vi "OpenFiles.vi"() -> ()   [LabVIEW 2018]
uses:
  <vilib>/addons/h5labview2/file/H5Fmode.ctl
  HDF5/HDF5_NoiseInfoClust.ctl
  HDF5/lib_path_mod_20200519.vi
  <vilib>/addons/h5labview2/base/H5Equery.vi
  <vilib>/addons/h5labview2/dataset/H5Dread.llb/H5Dread.xnode
  <vilib>/addons/h5labview2/file/H5F.lvlib
  <vilib>/addons/h5labview2/group/H5G.lvlib
panel:
  in  "Tree":string(tree)
  out "Folders":path[](array[path])
  out "Groups":string[](array[string])
  in  "Select 2":bool
  in  "Listbox 2":i32[](listbox)
  in  "Select":bool
  in  "Listbox":i32[](listbox)
  out "filenames":string[](array[string])
  in  "path":path
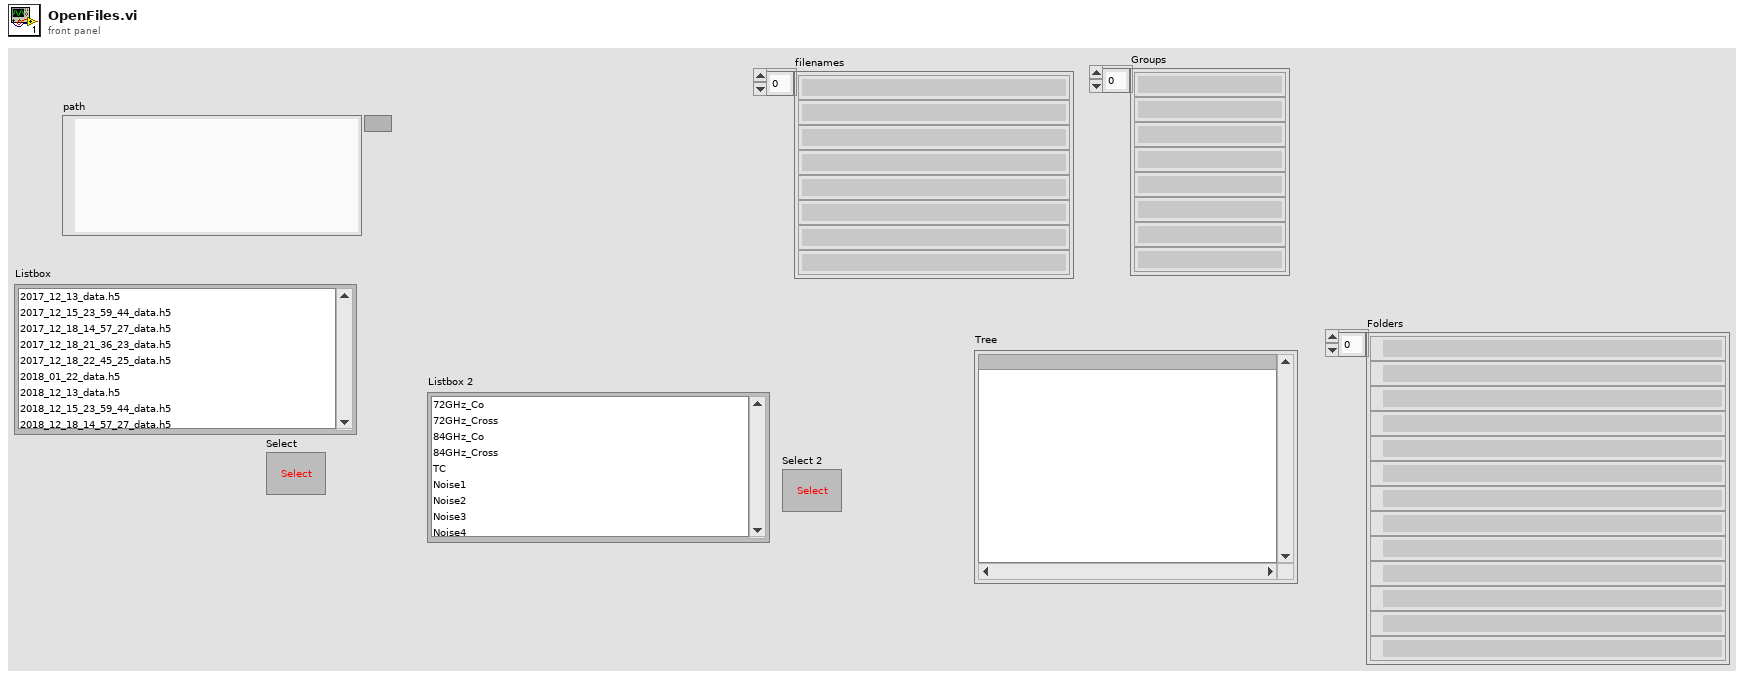
[diagram p1: front panel]
types:
  T1 = typedef "H5F.lvlib/H5Fmode.ctl" = enum16{"read-only", "read-write", "overwrite", "create new", "open or create"}
  T2 = typedef "hid_t.ctl" = i32
  T3 = typedef "HDF5_NoiseInfoClust.ctl" = cluster{"Timestring":string, "Timestamp":dbl, "df":dbl, "Sum":dbl}
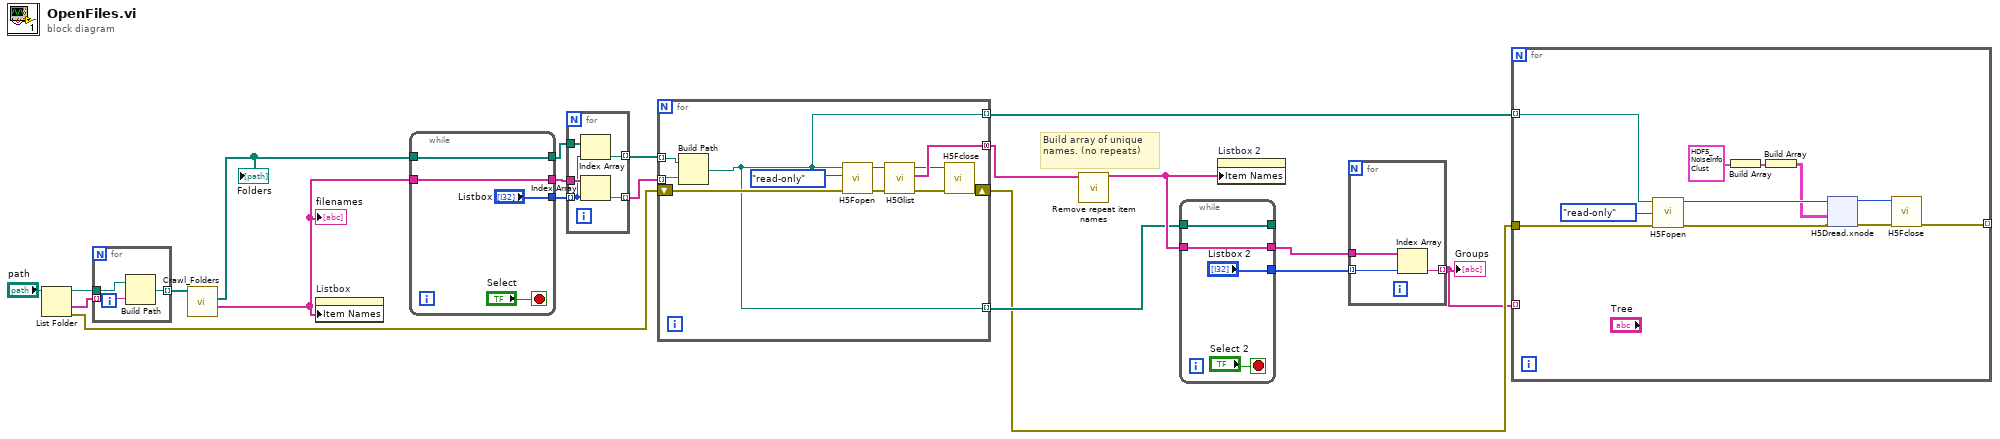
[diagram p0: block diagram]
diagram:
  # "Build array of unique names. (no repeats)"
  n1 = List Folder(path="path") -> (path out=w7:path, folder names=w8:string[], error out=w5:errorcluster)  [unwired: 3 in, 1 out]
  n2 = for {
    tunnel: w8 -> [w23] mode=indexing
    tunnel: w7 -> [w22]
    tunnel: [w21] -> w6 mode=indexing
    n3 = Build Path(base path=w22, name or relative path=w23) -> (appended path=w21:path)
  }
  n4 = call "Crawl_Folders.vi"("path in"=w6) -> ("FileNames"=w10:string[], "Folders"=w9:path[])  [unwired: 9 in]
  "filenames" <- w10
  "Folders" <- w9
  n5 = property on="Listbox" class="LstBox (strict)"("Item Names"=w10) -> ()  [unwired: 2 in, 2 out]
  n6 = while {
    tunnel: [w27] -> w11
    tunnel: w9 -> [w27]
    tunnel: w10 -> [w26]
    tunnel: [w26] -> w20
    tunnel: ["Listbox"] -> w19
    stop <- "Select" stop-if-true
  }
  n7 = for {
    tunnel: w20 -> [w32]
    tunnel: w19 -> [w28] mode=indexing
    tunnel: [w31] -> w18 mode=indexing
    tunnel: w11 -> [w30]
    tunnel: [w29] -> w4 mode=indexing
    n8 = Index Array(array=w30, index=w28) -> (element=w29:path)
    n9 = Index Array(array=w32, index=w28) -> (element=w31:string)
  }
  n10 = for {
    tunnel: w4 -> [w43] mode=indexing
    tunnel: w18 -> [w42] mode=indexing
    tunnel: [w39] -> w17 mode=concatenating
    tunnel: [w34] -> w15 mode=indexing
    tunnel: [w34] -> w3 mode=indexing
    shift-right: [w33] -> w2
    shift-left: w5 -> [w35]
    n11 = Build Path(base path=w43, name or relative path=w42) -> (appended path=w34:path)
    n12 = call <vilib>:"H5Fopen.vi"("error in (no error)"=w35, "mode (read-only)"=H5Fmode."read-only" ("mode"), "path"=w34) -> ("error out"=w38:errorcluster, "ref out"=w40:T2)  [unwired: 7 in]
    n13 = call <vilib>:"H5Glist.vi"("error in (no error)"=w38, "ref in"=w40) -> ("error out"=w37:errorcluster, "names"=w39:string[], "ref out"=w36:T2)  [unwired: 6 in, 1 out]
    n14 = call <vilib>:"H5Fclose.vi"("error in (no error)"=w37, "ref"=w36) -> ("error out"=w33:errorcluster)  [unwired: 9 in]
  }
  n15 = call "Remove repeat item names.vi"("names"=w17) -> ("Array"=w16:string[])  [unwired: 10 in]
  n16 = while {
    tunnel: [w47] -> _
    tunnel: w15 -> [w47]
    tunnel: w16 -> [w46]
    tunnel: [w46] -> w14
    tunnel: ["Listbox 2"] -> w13
    stop <- "Select 2" stop-if-true
  }
  n17 = property on="Listbox 2" class="LstBox (strict)"("Item Names"=w16) -> ()  [unwired: 2 in, 2 out]
  n18 = for {
    tunnel: w14 -> [w50]
    tunnel: w13 -> [w49] mode=indexing
    tunnel: [w48] -> w1 mode=indexing
    n19 = Index Array(array=w50, index=w49) -> (element=w48:string)
  }
  "Groups" <- w1
  n20 = for {
    tunnel: w3 -> [w60] mode=indexing
    tunnel: w2 -> [w58]
    tunnel: w1 -> [_] mode=indexing
    tunnel: [w52] -> _ mode=indexing
    n21 = call <vilib>:"H5Fopen.vi"("error in (no error)"=w58, "mode (read-only)"=H5Fmode."read-only" ("mode"), "path"=w60) -> ("error out"=w57:errorcluster, "ref out"=w59:T2)  [unwired: 7 in]
    n22 = Build Array(T3 {"Timestring"="Timestamp string goes here", "Timestamp"=0.0, "df"=7629.39453125, "Sum"=0.0} ("HDF5_NoiseInfo")) -> (w56:T3[])
    n23 = Build Array(w56) -> (w55:T3[][])
    n24 = xnode "H5Dread.xnode"("error in (no error)"=w57, "default"=w55, "ref in"=w59) -> ("error out"=w53:errorcluster, "ref out"=w51:i32)  [unwired: 3 in, 2 out]
    n25 = call <vilib>:"H5Fclose.vi"("error in (no error)"=w53, "ref"=w51) -> ("error out"=w52:errorcluster)  [unwired: 9 in]
  }
